vi "SHA-1.vi"(1 "Data":u8[](array[numeric])) -> (0 "output":string)   [LabVIEW 2017]
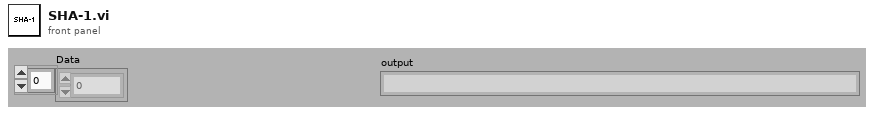
[diagram p1: front panel]
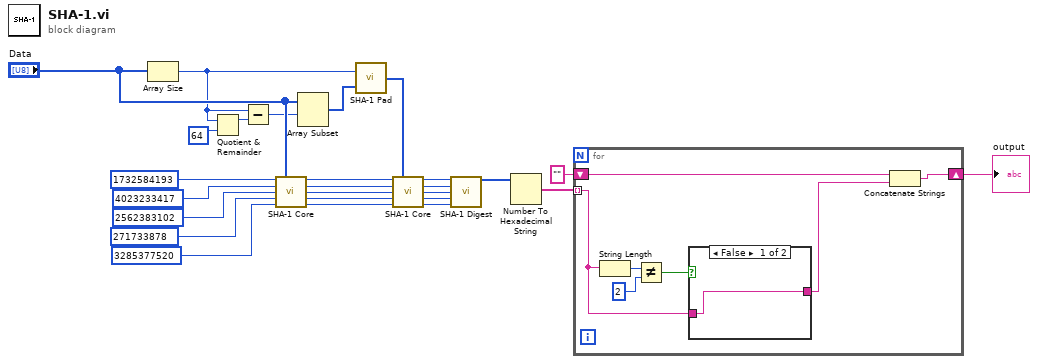
[diagram p0: block diagram]
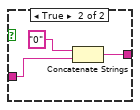
[diagram p2: hidden frame]
diagram:
  n1 = Array Size(array="Data") -> (size(s)=w5:i32)
  n2 = Quotient & Remainder(x=w5, y=64) -> (x-y*floor(x/y)=w16:i32)  [unwired: 1 out]
  n3 = Subtract(x=w5, y=w16) -> (x-y=w22:i32)
  n4 = call "SHA-1 Core.vi"("s1"=u32 1732584193, "Input Bytes"="Data", "s2"=u32 4023233417, "s3"=u32 2562383102, "s4"=u32 271733878, "s5"=u32 3285377520 ("s4")) -> ("s1 out"=w17:u32, "s2 out"=w18:u32, "s3 out"=w19:u32, "s4 out"=w20:u32, "s5 out"=w21:u32)  [unwired: 5 in]
  n5 = Array Subset(array="Data", index=w22) -> (w23:u8[])  [unwired: 1 in]
  n6 = call "SHA-1 Pad.vi"("Last Part"=w23, "Message Length (bytes)"=w5) -> ("Padding"=w24:u8[])
  n7 = call "SHA-1 Core.vi"("s1"=w17, "Input Bytes"=w24, "s2"=w18, "s3"=w19, "s4"=w20, "s5"=w21) -> ("s1 out"=w10:u32, "s2 out"=w9:u32, "s3 out"=w8:u32, "s4 out"=w7:u32, "s5 out"=w6:u32)  [unwired: 5 in]
  n8 = call "SHA-1 Digest.vi"("s1"=w10, "s2"=w9, "s3"=w8, "s4"=w7, "s5"=w6) -> ("message-digest"=w4:u8[])  [unwired: 10 in]
  n9 = Number To Hexadecimal String(2:w4) -> (0:w2:string[])  [unwired: 1 in]
  n10 = for {
    tunnel: w2 -> [w28] mode=indexing
    shift-right: [w33] -> w3
    shift-left: "" -> [w32]
    n11 = String Length(string=w28) -> (length=w31:i32)
    n12 = Not Equal?(x=w31, y=2) -> (x != y?=w29:bool)
    n13 = case shown="False" w29 {
      tunnel: w28 -> [w34 w36]
      tunnel: [w34 w35] -> w27
      frame False {
      }
      frame True {
        n14 = Concatenate Strings("0", w36) -> (w35:string)
      }
    }
    n15 = Concatenate Strings(w32, w27) -> (w33:string)
  }
  "output" <- w3
